vi "Stop Core.vi"(10 "final error code":i32, 11 "CS++DCPwr in":refnum<class "CS++DCPwr.lvclass">) -> (3 "CS++DCPwr out":refnum<class "CS++DCPwr.lvclass">)   [LabVIEW 2013, in "CS++DCPwr.lvlib" / "CS++DCPwr.lvclass"]
doc: "(<B>Filename</B>: Actor Framework.lvlib:Actor.lvclass:Stop Core.vi)\n\nDefines what the actor does before it stops. Use the <B>final error code</B> input to determine whether the actor shut down in response to an error.\n\nBy default, this method does nothing. A descendant class may override it to define behavior, such as shutting down any processes the actor initiated in its override of the Actor Core method."
uses:
  CS++DCPwr.lvclass
  <vilib>/ActorFramework/Time-Delayed Send Message/Time-Delay Override Options.ctl
  Core/Actors/CS++DeviceActor/CS++DeviceActor.lvclass
  CS++DCPwr.lvclass/CS++DCPwr.ctl
  Core/Classes/CS++ProcessVariables/PVConnection/PVConnection.lvclass
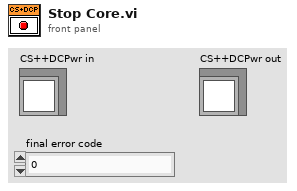
[diagram p1: front panel]
types:
  T1 = typedef "Time-Delay Override Options.ctl" = enum16{"Send next copy now", "Skip next scheduled copy", "Send next copy now and stop all further copies", "Stop all further copies"}
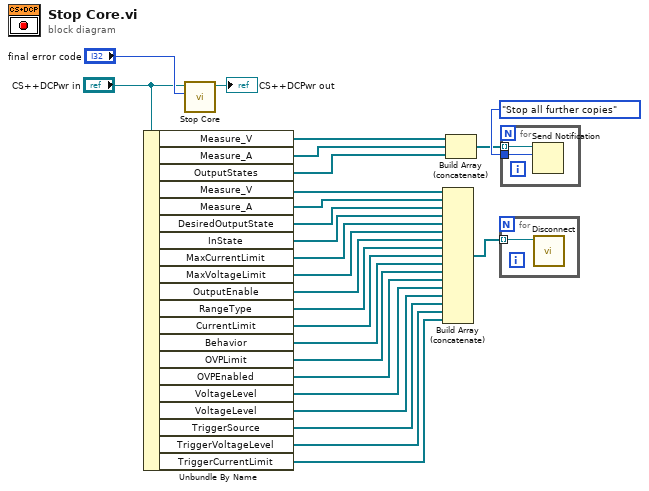
[diagram p0: block diagram]
diagram:
  n1 = Unbundle By Name("CS++DCPwr in") -> ("Measure_V"=w23:refnum<notifier>[], "Measure_A"=w19:refnum<notifier>[], "OutputStates"=w15:refnum<notifier>[], "Measure_V"=w22:refnum<class "PVConnection.lvclass">[], "Measure_A"=w17:refnum<class "PVConnection.lvclass">[], "DesiredOutputState"=w16:refnum<class "PVConnection.lvclass">[], "InState"=w14:refnum<class "PVConnection.lvclass">[], "MaxCurrentLimit"=w13:refnum<class "PVConnection.lvclass">[], "MaxVoltageLimit"=w12:refnum<class "PVConnection.lvclass">[], "OutputEnable"=w11:refnum<class "PVConnection.lvclass">[], "RangeType"=w10:refnum<class "PVConnection.lvclass">[], "CurrentLimit"=w9:refnum<class "PVConnection.lvclass">[], "Behavior"=w8:refnum<class "PVConnection.lvclass">[], "OVPLimit"=w7:refnum<class "PVConnection.lvclass">[], "OVPEnabled"=w6:refnum<class "PVConnection.lvclass">[], "VoltageLevel"=w5:refnum<class "PVConnection.lvclass">[], "VoltageLevel"=w4:refnum<class "PVConnection.lvclass">[], "TriggerSource"=w3:refnum<class "PVConnection.lvclass">[], "TriggerVoltageLevel"=w2:refnum<class "PVConnection.lvclass">[], "TriggerCurrentLimit"=w1:refnum<class "PVConnection.lvclass">[])
  n2 = call-parent "Stop Core.vi"("final error code"="final error code", "CS++DeviceActor in"="CS++DCPwr in") -> ("CS++DeviceActor out"=→"CS++DCPwr out":refnum<class "CS++DCPwr.lvclass">)  [unwired: 9 in]
  n3 = Build Array (concatenate)(w22, w17, w16, w14, w13, w12, w11, w10, w9, w8, w7, w6, w5, w4, w3, w2, w1) -> (w18:refnum<class "PVConnection.lvclass">[])
  n4 = Build Array (concatenate)(w23, w19, w15) -> (w20:refnum<notifier>[])
  n5 = for {
    tunnel: w18 -> [w27] mode=indexing
    n6 = call-dynamic "Disconnect.vi"("PVConnection in"=w27) -> ()  [unwired: 9 in, 2 out]
  }
  n7 = for {
    tunnel: w20 -> [w29] mode=indexing
    tunnel: Time-Delay_Override_Options."Stop all further copies" ("notification") -> [w28]
    n8 = Send Notification(notification=w28, notifier=w29) -> ()  [unwired: 1 in, 2 out]
  }
